vi "ConcatenateSweepResults.vi"(8 "error in (no error)":errorcluster, 9 "SweepResults [i]":T1, 10 "SweepResults []":T1, 11 "LockinDAQ":refnum<class "Instrument.DAQ.lvclass">) -> (0 "error out":errorcluster, 2 "SweepResults [] out":T1, 3 "LockinDAQ out":refnum<class "Instrument.DAQ.lvclass">)   [LabVIEW 2019, in "Instrument.DAQ.lvclass"]
uses:
  Instrument.DAQ.lvclass
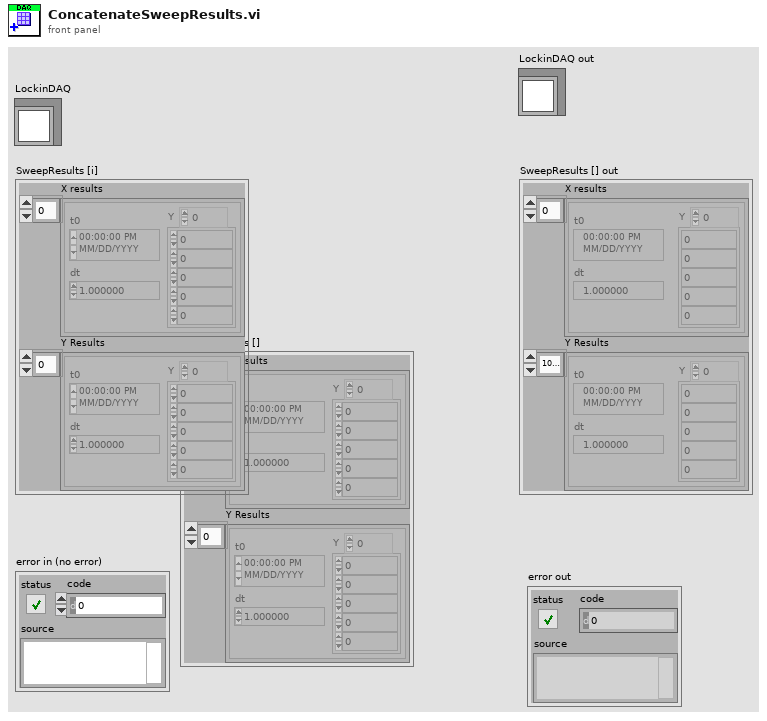
[diagram p1: front panel]
types:
  T1 = cluster{"X results":waveform(dbl)[], "Y Results":waveform(dbl)[]}
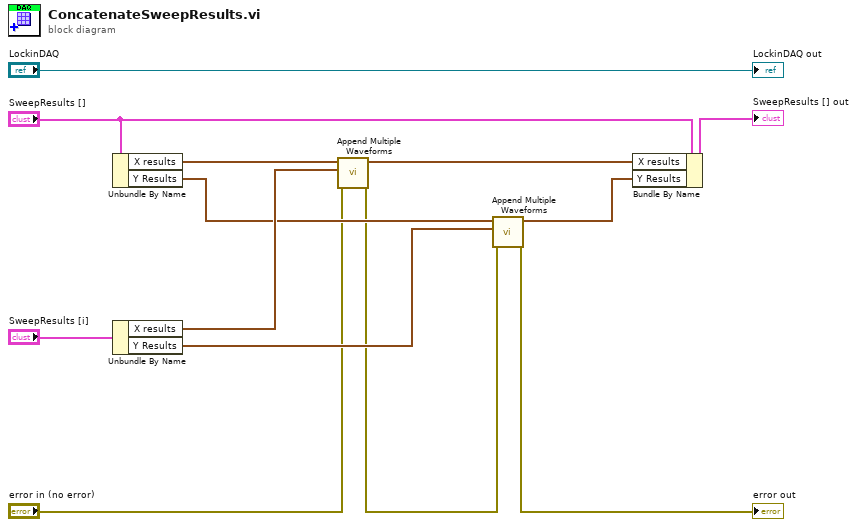
[diagram p0: block diagram]
diagram:
  n1 = Unbundle By Name("SweepResults []") -> ("X results"=w9:waveform(dbl)[], "Y Results"=w7:waveform(dbl)[])
  n2 = Unbundle By Name("SweepResults [i]") -> ("X results"=w8:waveform(dbl)[], "Y Results"=w6:waveform(dbl)[])
  n3 = call "Append Multiple Waveforms.vi"("error in (no error)"="error in (no error)", "Waveform B []"=w8, "Waveforrm A []"=w9) -> ("error out"=w4:errorcluster, "Waveform out []"=w2:waveform(dbl)[])  [unwired: 7 in]
  n4 = call "Append Multiple Waveforms.vi"("error in (no error)"=w4, "Waveform B []"=w6, "Waveforrm A []"=w7) -> ("error out"=→"error out":errorcluster, "Waveform out []"=w1:waveform(dbl)[])  [unwired: 7 in]
  n5 = Bundle By Name(cluster="SweepResults []", "X results"=w2, "Y Results"=w1) -> (→"SweepResults [] out":T1)
  "LockinDAQ out" <- "LockinDAQ"
